vi "Analyzer_Tester.vi"() -> ()   [LabVIEW 2012]
uses:
  <vilib>/addons/Wavelet Analysis/typedefs.llb/WA Data.ctl
  <vilib>/addons/_Advanced Signal Processing/NI_AdvSigProcWA.lvlib
panel:
  in  "Decomposition Level":i32=3
  in  "Wavelet":u16(ring) items=["db02"=0, "db03"=1, "db04"=2, "db05"=3, "db06"=4, "db07"=5, "db08"=6, "db09"=7, "db10"=8, "db11"=9, "db12"=10, "db13"=11, "db14"=12, "Haar"=13, "bior1_3"=14, "bior1_5"=15, "bior2_2"=16, "bior2_4"=17, "bior2_6"=18, "bior2_8"=19, "bior3_1"=20, "bior3_3"=21, "bior3_5"=22, "bior3_7"=23, "bior3_9"=24, "bior4_4 (FBI)"=25, "bior5_5"=38, "bior6_8"=39, "coif1"=26, "coif2"=27, "coif3"=28, "coif4"=29, "coif5"=30, "sym2"=31, "sym3"=32, "sym4"=33, "sym5"=34, "sym6"=35, "sym7"=36, "sym8"=37]
  in  "SigName":string="probnyEKG"
  out "Dets Graph":waveform(dbl)[](graph)
  out "Approx Graph":waveform(dbl)[](graph)
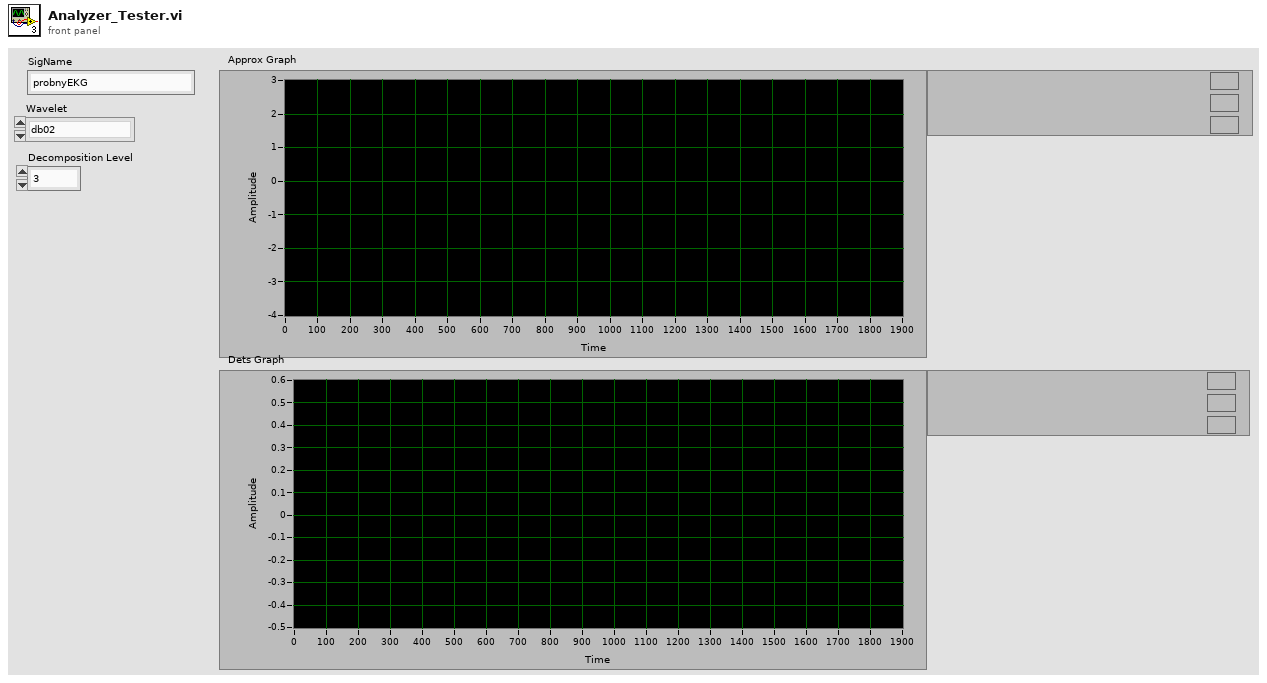
[diagram p1: front panel]
types:
  T1 = typedef "NI_AdvSigProcWA.lvlib/WA Data.ctl" = u16
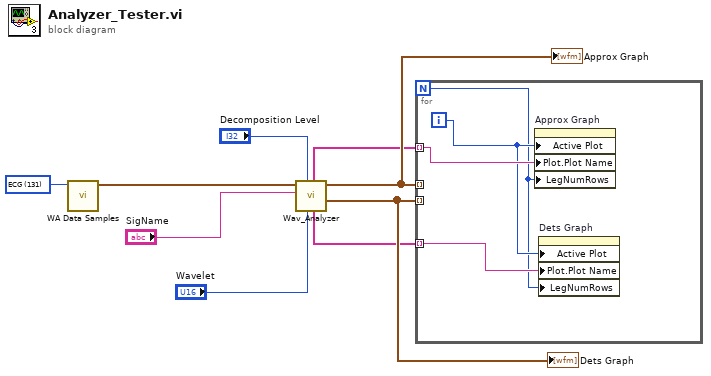
[diagram p0: block diagram]
diagram:
  w9 = T1 131 items=["1D Example Data"=100, "-"=101, "Doppler"=102, "HOP"=103, "TF Sine"=104, "Noisy Doppler"=105, "Sea Temperature"=106, "Sp500"=107, "Power Line"=108, "Engine Knocking"=109, "HeaviSine"=110, "Bumps"=111, "Blocks"=112, "Piece Regular"=113, "HypChirps"=114, "LinChirps"=115, "Chirps"=116, "Piece Polynomial"=117, "ECG"=131, "-"=118, "2D Example Data"=119, "-"=120, "Finger Print (Image)"=121, "Iris Flower (Image)"=122, "Mammogram (Image)"=123, "Lake (Image)"=127, "Two Can 1 (Image)"=132, "Two Can 2 (Image)"=133, "Camera Man (Image)"=134] ("data")
  n1 = call <vilib>:"WA Data Samples.vi"("data"=w9) -> ("signal"=w8:waveform(dbl))  [unwired: 9 in, 1 out]
  n2 = call "Wav_Analyzer.vi"("Wavelet"="Wavelet", "Decomposition Level"="Decomposition Level", "SigName"="SigName", "Signal"=w8) -> ("DetsArr"=w3:waveform(dbl)[], "ApproxArr"=w4:waveform(dbl)[], "DetsNArr"=w1:string[], "ApproxNArr"=w2:string[])  [unwired: 3 in, 1 out]
  "Approx Graph" <- w4
  "Dets Graph" <- w3
  n3 = for {
    N -> [w10]
    tunnel: w4 -> [_] mode=indexing
    tunnel: w3 -> [_] mode=indexing
    tunnel: w2 -> [w13] mode=indexing
    tunnel: w1 -> [w12] mode=indexing
    i -> [w11]
    n4 = property on="Approx Graph" class="WFGraph (strict)"("Active Plot"=w11, "Plot.Plot Name"=w13, "LegNumRows"=w10) -> ()  [unwired: 2 in, 2 out]
    n5 = property on="Dets Graph" class="WFGraph (strict)"("Active Plot"=w11, "Plot.Plot Name"=w12, "LegNumRows"=w10) -> ()  [unwired: 2 in, 2 out]
  }
